vi "Set Channel Resistance.vi"(8 "error in (no error)":errorcluster, 10 "Params":variant, 11 "PIPX40 Resistor in":refnum<class "PIPX40 Resistor.lvclass">) -> (0 "error out":errorcluster, 3 "PIPX40 Resistor out":refnum<class "PIPX40 Resistor.lvclass">)   [LabVIEW 2020, in "Pickering.lvlib" / "PIPX40 Resistor.lvclass"]
uses:
  PIPX40 Resistor.lvclass
  D:/WSGitHub/RTFWK/Realization/PIPX40 Base/PIPX40 Base.lvclass
  TypeDefs/Resistor channel.ctl
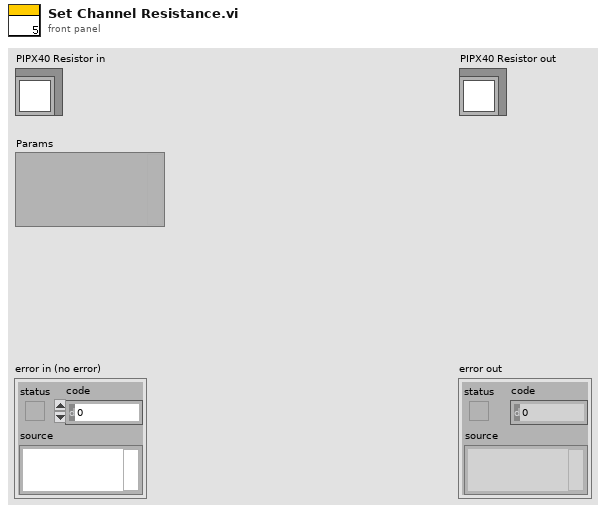
[diagram p1: front panel]
types:
  T1 = typedef "Pickering.lvlib/PIPX40 Resistor.lvclass/Resistor channel.ctl" = cluster{"subunit number":u32, "resistance":u16}
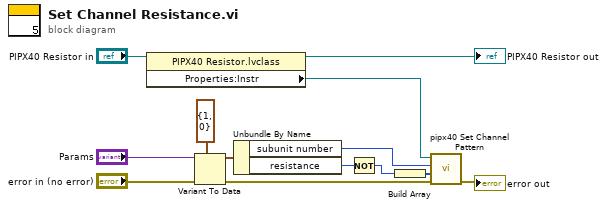
[diagram p0: block diagram]
diagram:
  n1 = property class="PIPX40 Resistor.lvclass"(reference="PIPX40 Resistor in") -> (reference out=→"PIPX40 Resistor out":refnum<class "PIPX40 Resistor.lvclass">, "Properties:Instr"=w10:refnum<visa-resource-name>)  [unwired: 1 in, 1 out]
  n2 = Variant To Data(error in="error in (no error)", type=T1 {"subunit number"=1, "resistance"=0}, Variant="Params") -> (data=w5:T1, error out=w9:errorcluster)
  n3 = Unbundle By Name(w5) -> ("subunit number"=w4:u32, "resistance"=w3:u16)
  n4 = Not(x=w3) -> (.not. x?=w2:u16)
  n5 = Build Array(w2) -> (w1:u16[])
  n6 = call <instrlib>:"pipx40 Set Channel Pattern.vi"("error in (no error)"=w9, "pattern"=w1, "subunit number"=w4, "instrument handle"=w10) -> ("error out"=→"error out":errorcluster)  [unwired: 6 in, 1 out]
